vi "Get Bit Value.vi"(7 "BitPosition":T1(ring), 10 "Data In":u8 format="%08b") -> (2 "BitValue":bool, 5 "BitValue(int)":u8 format="%08b")   [LabVIEW 2011]
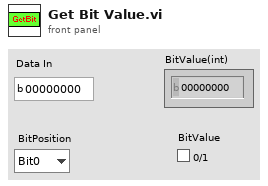
[diagram p1: front panel]
types:
  T1 = enum16{"Bit0", "Bit1", "Bit2", "Bit3", "Bit4", "Bit5", "Bit6", "Bit7"}
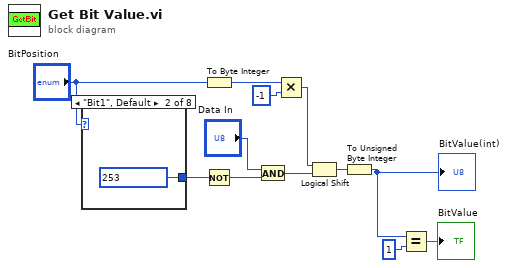
[diagram p0: block diagram]
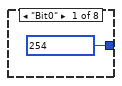
[diagram p2: hidden frame]
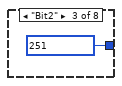
[diagram p3: hidden frame]
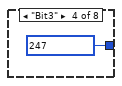
[diagram p4: hidden frame]
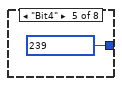
[diagram p5: hidden frame]
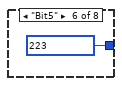
[diagram p6: hidden frame]
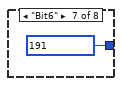
[diagram p7: hidden frame]
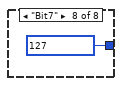
[diagram p8: hidden frame]
diagram:
  n1 = case shown="\"Bit1\", Default" "BitPosition" {
    tunnel: [u8 254 ("Data") u8 253 ("Data") u8 251 ("Data") u8 247 ("Data") u8 239 ("Data") u8 223 ("Data") u8 191 ("Data") u8 127 ("Data")] -> w12
    frame "Bit0" {
    }
    frame "Bit1", Default {
    }
    frame "Bit2" {
    }
    frame "Bit3" {
    }
    frame "Bit4" {
    }
    frame "Bit5" {
    }
    frame "Bit6" {
    }
    frame "Bit7" {
    }
  }
  n2 = To Byte Integer(number="BitPosition") -> (8bit integer=w7:i8)
  n3 = Not(x=w12) -> (.not. x?=w4:u8)
  n4 = And(x="Data In", y=w4) -> (x .and. y?=w10:u8)
  n5 = Multiply(x=w7, y=i8 -1) -> (x*y=w6:i8)
  n6 = Logical Shift(y=w6, x=w10) -> (x << y=w11:u8)
  n7 = To Unsigned Byte Integer(number=w11) -> (unsigned 8bit integer=w3:u8)
  "BitValue(int)" <- w3
  n8 = Equal?(x=w3, y=u8 1) -> (x = y?=→"BitValue":bool)
